vi "HighLvCtrl_Loop_Squat.vi"(8 "error in (no error)":errorcluster, 11 "HighLvClasses":T4={"CAlexVersion"=enum."Mobile", "CAlex2 out"=refnum, "ForceField"=refnum}) -> (0 "error out":errorcluster)   [LabVIEW 2016]
uses:
  <vilib>/Platform/TimedLoop/XDataNode/wakeup.ctl
  <vilib>/Platform/TimedLoop/XDataNode/XDNodeRunTimeDep.lvlib
  <vilib>/Platform/TimedLoop/XDataNode/nitl_modes.ctl
  <vilib>/Platform/TimedLoop/XDataNode/timing_clust.ctl
  <vilib>/Platform/TimedLoop/XDataNode/XDataNode.xnode
  Classes/SerialChain/SerialChain.lvclass
  Classes/SerialChain-Cable/SerialChain-Cable.lvclass
  Classes/ForceField/ForceField.lvclass
  <vilib>/Analysis/NI_AALBase.lvlib
  <vilib>/Analysis/Matrix/Datatypes/RealMatrix.ctl
  <vilib>/Analysis/Matrix/NI_Matrix.lvlib
  <vilib>/AuZn/auzn custom VIs/AuZnCustomVI.lvlib
  Classes/CAlex2/CAlex2.lvclass
  TypeDef/IMU_operation.ctl
  <vilib>/Analysis/baseanly.llb/A x Vector.vi
  C:/Users/randh/Desktop/BILATERAL/CAlex2-controller/Classes/SerialChain-Cable/SerialChain-Cable.lvclass
  C:/Users/randh/Desktop/BILATERAL/CAlex2-controller/Classes/SerialChain/SerialChain.lvclass
  Classes/ForceField/TypeDef/FF_Gains.ctl
  Classes/CAlex2/TypeDef/LowerBodyDim.ctl
  Classes/MotorControl/TypeDef/ControllerMode.ctl
  TypeDef/HighLvControl Cluster.ctl
  Classes/CAlex2/TypeDef/CAlexVersion.ctl
panel:
  in  "Use Vicon2JointAngle2 ?":bool=TRUE
  in  "Use IMU2JointAngle2 ?":bool=TRUE
  in  "history length (50)":i32=50
  in  "LP":bool=TRUE
  out "QPSolved":bool
  out "Torque Error":dbl[](array[numeric]) format="%#.4f"
  out "Torque":T1(graph)
  out "Joint Angles (deg)":T2(graph)
  out "Desired Torque":dbl[](array[numeric]) format="%#.4f"
  out "Actual Torque":dbl[](array[numeric]) format="%#.4f"
  in  "LockedJoints":i32[](array[numeric])=[2, 1]
  out "Jacobian for Cables":T3 format="%#.3f"
  in  "TargetF(N)":dbl=10.0 format="%#_13g"
  in  "LP fc":dbl=4.0 format="%0.3f"
  in  "QPmode":enum16{"tight", "loose", "adv"}(ring)=enum."adv"
  in  "F range":cluster{"Fmin":dbl, "Fmax":dbl}[](array[cluster])=[{"Fmin"=10.0, "Fmax"=80.0}, {"Fmin"=10.0, "Fmax"=80.0}, {"Fmin"=11.0, "Fmax"=80.0}, {"Fmin"=11.0, "Fmax"=80.0}]
  # "In Cable Order, Not Motor Order"
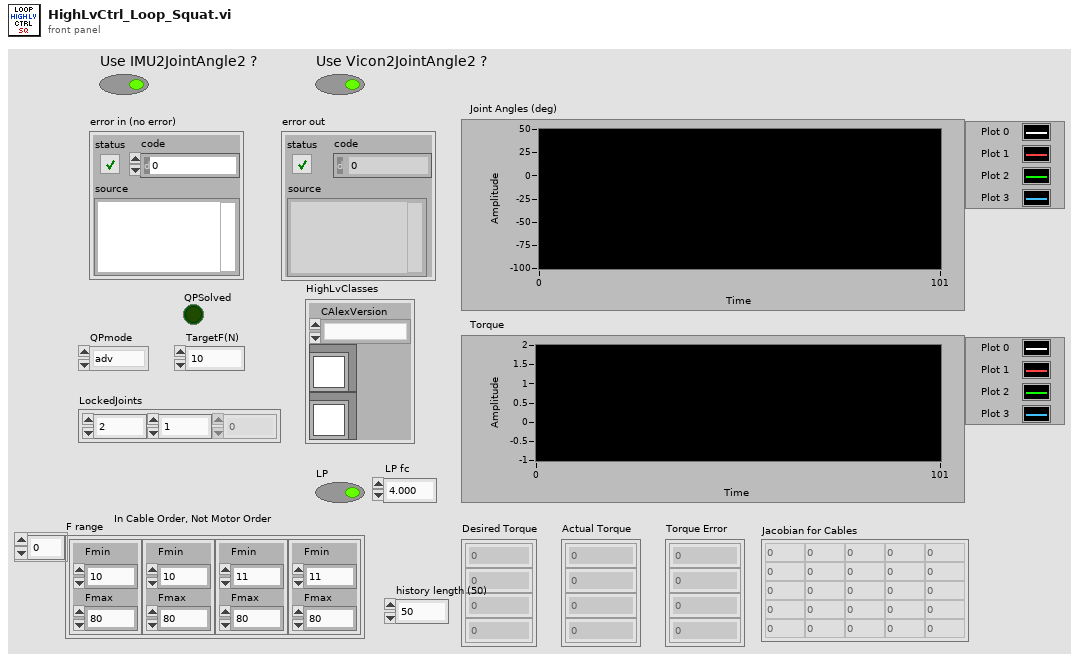
[diagram p1: front panel]
types:
  T1 = cluster{"[0]":dbl, "[1]":dbl, "[2]":dbl, "[3]":dbl, "[4]":dbl, "[5]":dbl, "[6]":dbl, "[7]":dbl, "[8]":dbl}
  T2 = cluster{"Joint Angles (rad)[0]":dbl, "Joint Angles (rad)[1]":dbl, "Joint Angles (rad)[2]":dbl, "Joint Angles (rad)[3]":dbl}
  T3 = typedef "NI_Matrix.lvlib/RealMatrix.ctl" = dbl[][]
  T4 = typedef "HighLvControl Cluster.ctl" = cluster{"CAlexVersion":T5, "CAlex2 out":refnum<class "CAlex2.lvclass">, "ForceField":refnum<class "ForceField.lvclass">}
  T5 = typedef "CAlex2.lvclass/CAlexVersion.ctl" = enum16{"Bilateral", "Squat", "Bilateral_Squat", "Treadmill", "Mobile"}
  T6 = typedef "XDNodeRunTimeDep.lvlib/timing_clust.ctl" = cluster{"Expected End [f-1]":u64, "Actual End [f-1]":u64, "Finished Late? [f-1]":bool, "Expected End [i-1]":u64, "Actual End [i-1]":u64, "Finished Late? [i-1]":bool, "Expected Start [i]":u64, "Actual Start [i]":u64, "Expected Start [f]":u64, "Actual Start [f]":u64, "Source Name":string, "Structure Name":string, "Period":i64, "Deadline":i64, "Offset":i64, "Start":i64, "Priority":i32, "Timeout":i32, "Mode":T7, "Wakeup Reason":T8, "Error":errorcluster, "Source Type":string, "Secondary Source Type":string, "Global End Time":u64, "Global Start Time":u64, "Frame Duration":u64, "Iteration Duration":u64, "Assigned CPU":i32, "I/O Scan Engine Mode":u32}
  T7 = typedef "XDNodeRunTimeDep.lvlib/nitl_modes.ctl" = enum32{"No Change", "Process missed periods, maintain original phase", "Discard missed periods, maintain original phase", "Process missed periods, ignore original phase", "Discard missed periods, ignore original phase"}
  T8 = typedef "XDNodeRunTimeDep.lvlib/wakeup.ctl" = enum32{"Normal", "Aborted", "Asynchronous wakeup", "Timing source error", "Timed loop error", "Timeout"}
  T9 = typedef "IMU_operation.ctl" = enum16{"GetData", "ClearStandPos", "SetStandPos"}
  T10 = typedef "ForceField.lvclass/FF_Gains.ctl" = cluster{"Kn":dbl, "Dn":dbl, "Kt":dbl, "Dt":dbl, "Kd":dbl, "Ns":dbl}
  T11 = typedef "CAlex2.lvclass/LowerBodyDim.ctl" = cluster{"BodyDim":cluster{"ThighLt (m)":dbl, "ShankLt (m)":dbl, "HipWd (m)":dbl}, "BodyWt":cluster{"Thigh (kg)":dbl, "Shank (kg)":dbl}, "Cuff Loc":cluster{"HipCuffWd (m)":dbl, "HipCuffHt (m)":dbl, "HipFwdShift (m)":dbl, "ThighToKnee (m)":dbl, "ThighCuffDist (m)":dbl, "ShankToKnee (m)":dbl}}
  T12 = typedef "SerialChain.lvclass/PointOnBody.ctl" = cluster{"Coord4":dbl[], "ID":i32}
  T13 = typedef "MotorControl.lvclass/ControllerMode.ctl" = enum16{"Idle", "FF", "PID"}
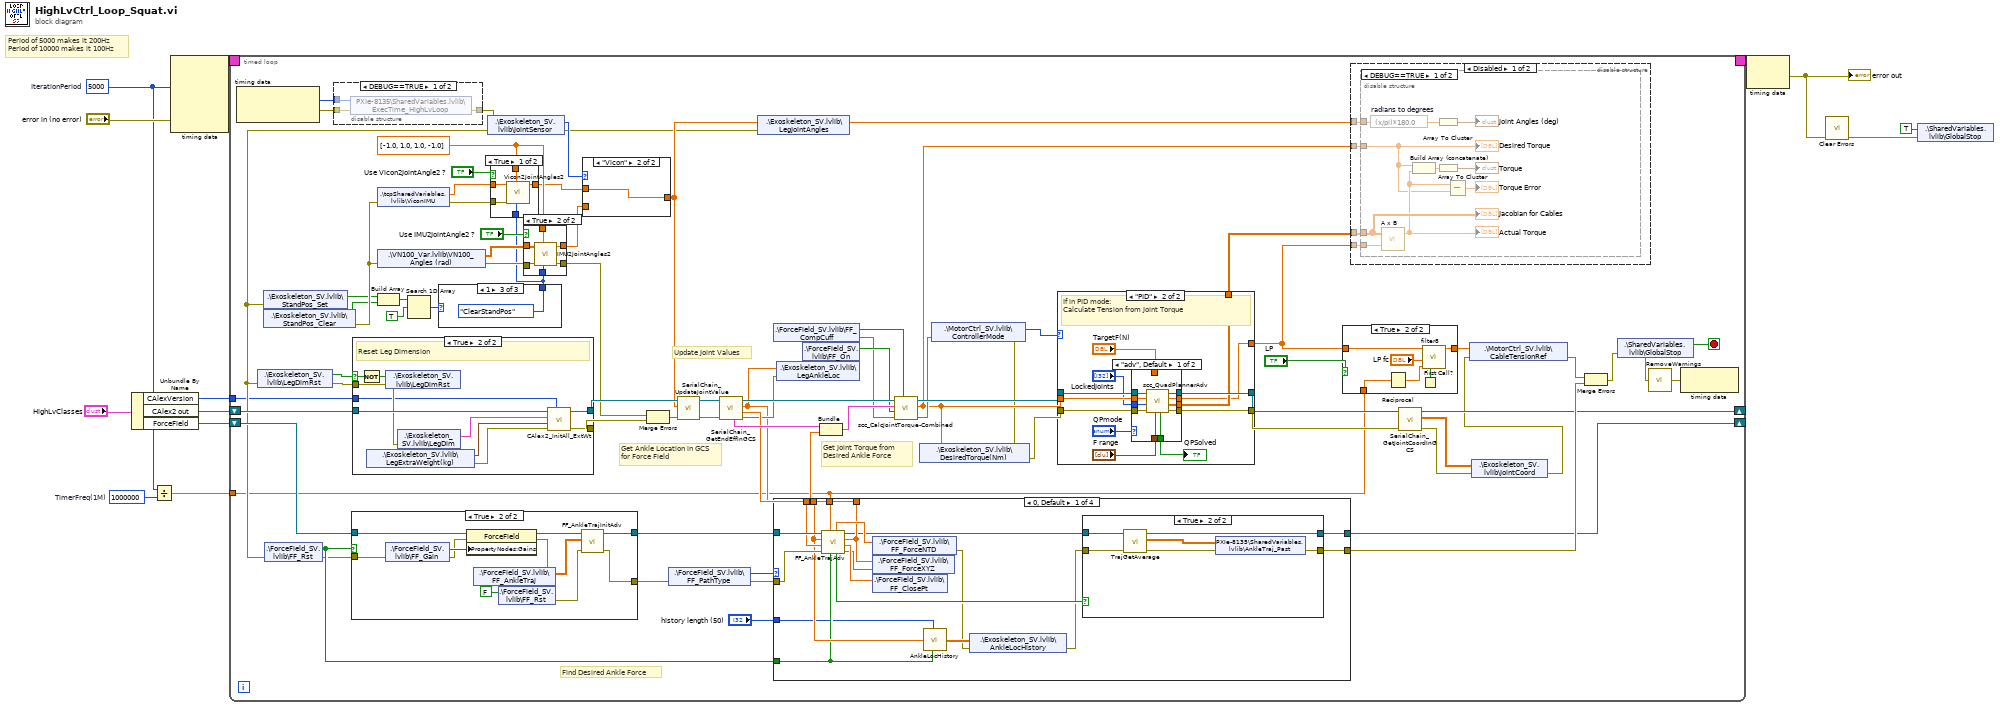
[diagram p0: block diagram]
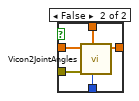
[diagram p5: hidden frame]
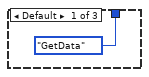
[diagram p6: hidden frame]
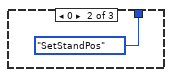
[diagram p7: hidden frame]
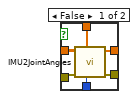
[diagram p8: hidden frame]
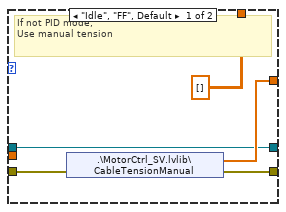
[diagram p11: hidden frame]
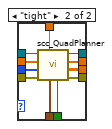
[diagram p12: hidden frame]
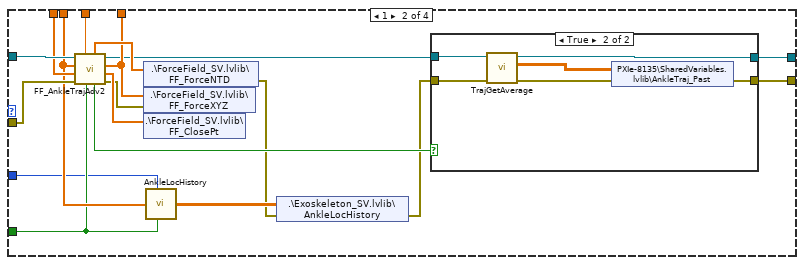
[diagram p16: hidden frame]
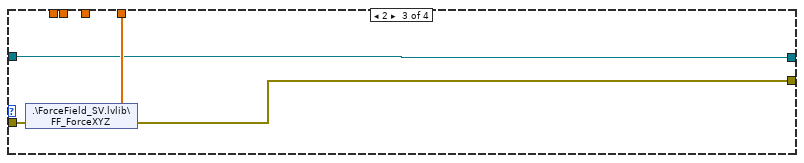
[diagram p18: hidden frame]
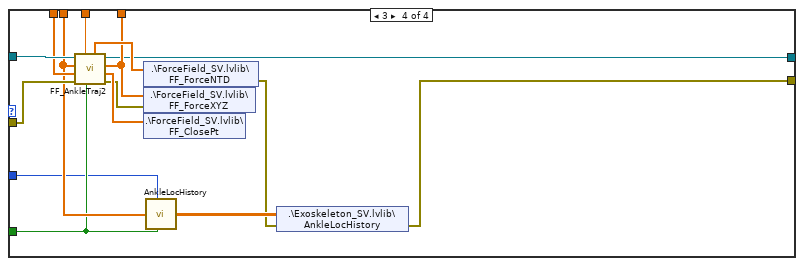
[diagram p19: hidden frame]
diagram:
  w3 = i64 1000000  # TimerFreq(1M)
  w4 = i64 5000  # IterationPeriod
  # "Period of 5000 makes it 200Hz\nPeriod of 10000 makes it 100Hz"
  n1 = Unbundle By Name("HighLvClasses") -> ("CAlexVersion"=w1:T5, "CAlex2 out"=w9:refnum<class "CAlex2.lvclass">, "ForceField"=w8:refnum<class "ForceField.lvclass">)
  n2 = Divide(x=w4, y=w3) -> (x/y=w2:dbl)
  n3 = node-c288(w4, "error in (no error)") -> (w13:T6)  [unwired: 3 in]
  n4 = timed-loop {
    timing: w13 -> [_]
    timing-out: [_] -> w12
    shift-right: [w47] -> _
    shift-left: w9 -> [w90]
    shift-right: [w60] -> _
    shift-left: w8 -> [w87]
    tunnel: w2 -> [w15]
    tunnel: w1 -> [w14]
    stop <- w62 stop-if-true
    w33 = dbl[] [-1.0, 1.0, 1.0, -1.0]
    # "Get Joint Torque from Desired Ankle Force"
    # "Find Desired Ankle Force"
    # "Get Ankle Location in GCS for Force Field"
    # "Update Joint Values"
    n5 = node-c288() -> (w89:i64, w88:errorcluster)  [unwired: 1 in]
    n6 = disable-structure shown="DEBUG==TRUE" {
      disable-tunnel: w89 -> [w141 _]
      disable-tunnel: w88 -> [w140 w142]
      disable-tunnel: [w139 w142] -> w17
      frame condition #0 {
        n7 = shared-variable "PXIe-8135\\SharedVariables.lvlib\\ExecTime_HighLvLoop"(w141, error in=w140) -> (error out=w139:errorcluster)
      }
      frame condition #1 (active) {
      }
    }
    n8 = shared-variable ".\\Exoskeleton_SV.lvlib\\LegDimRst"(error in=w17) -> (w71:bool, error out=w82:errorcluster)
    n9 = shared-variable ".\\Exoskeleton_SV.lvlib\\StandPos_Set"(error in=w17) -> (w25:bool, error out=w64:errorcluster)
    n10 = shared-variable ".\\Exoskeleton_SV.lvlib\\StandPos_Clear"(error in=w64) -> (w24:bool, error out=w32:errorcluster)
    n11 = shared-variable ".\\ForceField_SV.lvlib\\FF_Rst"(error in=w17) -> (w68:bool, error out=w67:errorcluster)
    n12 = case shown="True" w68 {
      tunnel: w87 -> [w182 w194]
      tunnel: [w182 w193] -> w81
      tunnel: w67 -> [w181 w189]
      tunnel: [w181 w183] -> w70
      frame False {
      }
      frame True {
        n13 = shared-variable ".\\ForceField_SV.lvlib\\FF_Gain"(error in=w189) -> (w192:T10, error out=w187:errorcluster)
        n14 = property class="ForceField"(reference=w194, error in=w187, "PropertyNodes:Gains"=w192) -> (reference out=w191:refnum<class "ForceField.lvclass">, error out=w186:errorcluster)
        n15 = shared-variable ".\\ForceField_SV.lvlib\\FF_AnkleTraj"(error in=w186) -> (w190:dbl[][], error out=w185:errorcluster)
        n16 = shared-variable ".\\ForceField_SV.lvlib\\FF_Rst"(FALSE ("FFRst"), error in=w185) -> (error out=w184:errorcluster)
        n17 = call "FF_AnkleTrajInitAdv.vi"("error in (no error)"=w184, "AnkleTraj"=w190, "Force Field Controller in"=w191) -> ("error out"=w183:errorcluster, "Force Field Controller out"=w193:refnum<class "ForceField.lvclass">)  [unwired: 6 in, 1 out]
      }
    }
    n18 = case shown="True" w71 {
      selector: w71 -> [_ w203]
      tunnel: w90 -> [w196 w208]
      tunnel: [w196 w207] -> w83
      tunnel: w82 -> [w195 w206]
      tunnel: [w195 w201] -> w39
      tunnel: w14 -> [_ w197]
      frame False {
      }
      frame True {
        # "Reset Leg Dimension"
        n19 = Not(x=w203) -> (.not. x?=w204:bool)
        n20 = shared-variable ".\\Exoskeleton_SV.lvlib\\LegDimRst"(w204, error in=w206) -> (error out=w200:errorcluster)
        n21 = shared-variable ".\\Exoskeleton_SV.lvlib\\LegDim"(error in=w200) -> (w205:T11, error out=w199:errorcluster)
        n22 = shared-variable ".\\Exoskeleton_SV.lvlib\\LegExtraWeight(kg)"(error in=w199) -> (w202:cluster{"Thigh":dbl, "Shank":dbl}, error out=w198:errorcluster)
        n23 = call "CAlex2_InitAll_ExtWt.vi"("CAlexVersion"=w197, "error in (no error)"=w198, "ExtraWeight(kg)"=w202, "LegProperties"=w205, "CAlex2 in"=w208) -> ("error out"=w201:errorcluster, "CAlex2 out"=w207:refnum<class "CAlex2.lvclass">)  [unwired: 5 in]
      }
    }
    n24 = shared-variable ".\\VN100_Var.lvlib\\VN100_Angles (rad)"(error in=w32) -> (w36:dbl[][], error out=w37:errorcluster)
    n25 = Build Array(w25, w24) -> (w23:bool[])
    n26 = shared-variable ".\\tcpSharedVariables.lvlib\\ViconIMU"(error in=w32) -> (w35:dbl[], error out=w34:errorcluster)
    n27 = Search 1D Array(1D array=w23, element=TRUE) -> (index of element=w22:i32)  [unwired: 1 in]
    n28 = case shown="1" w22 {
      tunnel: [IMU_operation."GetData" ("Operation(GetData)") IMU_operation."SetStandPos" ("Operation(GetData)") IMU_operation."ClearStandPos" ("Operation(GetData)")] -> w20
      frame Default {
      }
      frame 0 {
      }
      frame 1 {
      }
    }
    n29 = shared-variable ".\\Exoskeleton_SV.lvlib\\JointSensor"(error in=w17) -> (w31:enum16{"IMU", "Vicon"}, error out=w27:errorcluster)
    n30 = case shown="True" "Use Vicon2JointAngle2 ?" {
      tunnel: w35 -> [w116 w121]
      tunnel: w34 -> [w115 w120]
      tunnel: w33 -> [w114 w119]
      tunnel: [w113 w118] -> w30
      tunnel: w20 -> [w112 w117]
      frame True {
        n31 = call "Vicon2JointAngles2.vi"("Operation(GetData)"=w112, "JointAngleDir([-1,1,1,-1])"=w114, "error in (no error)"=w115, "ViconIMU in (rad)"=w116) -> ("Joint Angles (rad)"=w113:dbl[])  [unwired: 6 in, 1 out]
      }
      frame False {
        n32 = call "Vicon2JointAngles.vi"("Operation(GetData)"=w117, "JointAngleDir([-1,1,1,-1])"=w119, "error in (no error)"=w120, "ViconIMU in (rad)"=w121) -> ("Joint Angles (rad)"=w118:dbl[])  [unwired: 6 in, 1 out]
      }
    }
    n33 = case shown="True" "Use IMU2JointAngle2 ?" {
      tunnel: w37 -> [w130 w136]
      tunnel: w36 -> [w129 w135]
      tunnel: w33 -> [w128 w134]
      tunnel: [w127 w133] -> w29
      tunnel: w20 -> [w126 w132]
      tunnel: [w125 w131] -> w19
      frame False {
        n34 = call "IMU2JointAngles.vi"("Operation(GetData)"=w126, "JointAngleDir (-1, 1, 1,-1)"=w128, "error in (no error)"=w130, "IMU in (rad)"=w129) -> ("error out"=w125:errorcluster, "Joint Angles (rad)"=w127:dbl[])  [unwired: 6 in]
      }
      frame True {
        n35 = call "IMU2JointAngles2.vi"("Operation(GetData)"=w132, "JointAngleDir (-1, 1, 1,-1)"=w134, "error in (no error)"=w136, "IMU in (rad)"=w135) -> ("error out"=w131:errorcluster, "Joint Angles (rad)"=w133:dbl[])  [unwired: 6 in]
      }
    }
    n36 = case shown="\"Vicon\"" w31 {
      tunnel: w30 -> [_ w138]
      tunnel: [w137 w138] -> w28
      tunnel: w29 -> [w137 _]
      frame "IMU", Default {
      }
      frame "Vicon" {
      }
    }
    n37 = Merge Errors(w19, w39) -> (w38:errorcluster)
    n38 = shared-variable ".\\ForceField_SV.lvlib\\FF_PathType"(error in=w70) -> (w77:i8, error out=w76:errorcluster)
    n39 = call "SerialChain_UpdateJointValue.vi"("error in (no error)"=w38, "JointAngle (rad | m)"=w28, "SerialChain in"=w83) -> ("error out"=w50:errorcluster, "SerialChain out"=w51:refnum<class "CAlex2.lvclass">)  [unwired: 7 in]
    n40 = call "SerialChain_GetEndEffInGCS.vi"("error in (no error)"=w50, "SerialChain in"=w51) -> ("error out"=w69:errorcluster, "Vendeff(GCS)"=w78:dbl[], "Pendeff(GCS)"=w43:dbl[], "SerialChain out"=w85:refnum<class "CAlex2.lvclass">, "EndEffPos"=w86:T12)  [unwired: 5 in]
    n41 = shared-variable ".\\Exoskeleton_SV.lvlib\\LegJointAngles"(w28, error in=w27) -> ()  [unwired: 1 out]
    n42 = case shown="0, Default" w77 {
      tunnel: w81 -> [w228 w256 w267 w285]
      tunnel: w76 -> [w224 w252 w266 w281]
      tunnel: [w217 w245 w267 w271] -> w60
      tunnel: [w223 w251 w268 w280] -> w79
      tunnel: w43 -> [w213 w241 _ w274]
      tunnel: w78 -> [w220 w248 _ w277]
      tunnel: w15 -> [w219 w247 _ w276]
      tunnel: w68 -> [w212 w240 _ w273]
      tunnel: [w216 w244 w265 w270] -> w61
      tunnel: "history length (50)" -> [w209 w237 _ w269]
      frame 0, Default {
        n43 = call "FF_AnkleTrajAdv.vi"("Init"=w212, "dt"=w219, "error in (no error)"=w224, "AnkleVelocity"=w220, "AnkleInGCS"=w213, "Force Field Controller in"=w228) -> ("error out"=w222:errorcluster, "ClosestPoint"=w226:dbl[], "ForceXYZ"=w223:dbl[], "Force Field Controller out"=w218:refnum<class "ForceField.lvclass">, "UpdateTrajPrev"=w215:bool, "ForceNTD"=w227:dbl[])
        n44 = shared-variable ".\\ForceField_SV.lvlib\\FF_ForceXYZ"(w223, error in=w222) -> (error out=w221:errorcluster)
        n45 = shared-variable ".\\ForceField_SV.lvlib\\FF_ClosePt"(w226, error in=w221) -> (error out=w225:errorcluster)
        n46 = shared-variable ".\\ForceField_SV.lvlib\\FF_ForceNTD"(w227, error in=w225) -> (error out=w211:errorcluster)
        n47 = call "AnkleLocHistory.vi"("history length (100)"=w209, "AnkleLoc"=w213, "initialize"=w212) -> ("AnkleLoc"=w214:dbl[][])  [unwired: 2 in]
        n48 = shared-variable ".\\Exoskeleton_SV.lvlib\\AnkleLocHistory"(w214, error in=w211) -> (error out=w210:errorcluster)
        n49 = case shown="True" w215 {
          tunnel: w218 -> [w230 w235]
          tunnel: [w230 w236] -> w217
          tunnel: w210 -> [w229 w233]
          tunnel: [w229 w231] -> w216
          frame False {
          }
          frame True {
            n50 = call-dynamic "TrajGetAverage.vi"("error in (no error)"=w233, "ForceField in"=w235) -> ("error out"=w232:errorcluster, "Ankle Traj Ave"=w234:dbl[][], "ForceField out"=w236:refnum<class "ForceField.lvclass">)  [unwired: 7 in]
            n51 = shared-variable "PXIe-8135\\SharedVariables.lvlib\\AnkleTraj_Past"(w234, error in=w232) -> (error out=w231:errorcluster)
          }
        }
      }
      frame 1 {
        n52 = call "FF_AnkleTrajAdv2.vi"("Init"=w240, "dt"=w247, "error in (no error)"=w252, "AnkleVelocity"=w248, "AnkleInGCS"=w241, "Force Field Controller in"=w256) -> ("error out"=w250:errorcluster, "ClosestPoint"=w254:dbl[], "Assistive Force in GCS"=w251:dbl[], "Force Field Controller out"=w246:refnum<class "ForceField.lvclass">, "UpdateTrajAve"=w243:bool, "Assistive Force FnFtFd"=w255:dbl[])
        n53 = shared-variable ".\\ForceField_SV.lvlib\\FF_ForceXYZ"(w251, error in=w250) -> (error out=w249:errorcluster)
        n54 = shared-variable ".\\ForceField_SV.lvlib\\FF_ClosePt"(w254, error in=w249) -> (error out=w253:errorcluster)
        n55 = shared-variable ".\\ForceField_SV.lvlib\\FF_ForceNTD"(w255, error in=w253) -> (error out=w239:errorcluster)
        n56 = call "AnkleLocHistory.vi"("history length (100)"=w237, "AnkleLoc"=w241, "initialize"=w240) -> ("AnkleLoc"=w242:dbl[][])  [unwired: 2 in]
        n57 = shared-variable ".\\Exoskeleton_SV.lvlib\\AnkleLocHistory"(w242, error in=w239) -> (error out=w238:errorcluster)
        n58 = case shown="True" w243 {
          tunnel: w246 -> [w258 w263]
          tunnel: [w258 w264] -> w245
          tunnel: w238 -> [w257 w261]
          tunnel: [w257 w259] -> w244
          frame False {
          }
          frame True {
            n59 = call-dynamic "TrajGetAverage.vi"("error in (no error)"=w261, "ForceField in"=w263) -> ("error out"=w260:errorcluster, "Ankle Traj Ave"=w262:dbl[][], "ForceField out"=w264:refnum<class "ForceField.lvclass">)  [unwired: 7 in]
            n60 = shared-variable "PXIe-8135\\SharedVariables.lvlib\\AnkleTraj_Past"(w262, error in=w260) -> (error out=w259:errorcluster)
          }
        }
      }
      frame 2 {
        n61 = shared-variable ".\\ForceField_SV.lvlib\\FF_ForceXYZ"(error in=w266) -> (w268:dbl[], error out=w265:errorcluster)
      }
      frame 3 {
        n62 = call "FF_AnkleTraj2.vi"("Init"=w273, "dt"=w276, "error in (no error)"=w281, "AnkleVelocity"=w277, "AnkleInGCS"=w274, "Force Field Controller in"=w285) -> ("error out"=w279:errorcluster, "ClosePt"=w283:dbl[], "Force"=w280:dbl[], "Force Field Controller out"=w271:refnum<class "ForceField.lvclass">, "ForceComp"=w284:dbl[])  [unwired: 1 in]
        n63 = shared-variable ".\\ForceField_SV.lvlib\\FF_ForceXYZ"(w280, error in=w279) -> (error out=w278:errorcluster)
        n64 = shared-variable ".\\ForceField_SV.lvlib\\FF_ClosePt"(w283, error in=w278) -> (error out=w282:errorcluster)
        n65 = shared-variable ".\\ForceField_SV.lvlib\\FF_ForceNTD"(w284, error in=w282) -> (error out=w272:errorcluster)
        n66 = call "AnkleLocHistory.vi"("history length (100)"=w269, "AnkleLoc"=w274, "initialize"=w273) -> ("AnkleLoc"=w275:dbl[][])  [unwired: 2 in]
        n67 = shared-variable ".\\Exoskeleton_SV.lvlib\\AnkleLocHistory"(w275, error in=w272) -> (error out=w270:errorcluster)
      }
    }
    n68 = shared-variable ".\\Exoskeleton_SV.lvlib\\LegAnkleLoc"(w43, error in=w69) -> (error out=w74:errorcluster)
    n69 = shared-variable ".\\ForceField_SV.lvlib\\FF_On"(error in=w74) -> (w73:bool, error out=w75:errorcluster)
    n70 = shared-variable ".\\ForceField_SV.lvlib\\FF_CompCuff"(error in=w75) -> (w59:bool, error out=w72:errorcluster)
    n71 = Bundle("EndEffPos"=w86, "Force"=w79) -> (w80:cluster{"EndEffPos":T12, "Force":dbl[]})  [unwired: 1 in]
    n72 = call "scc_CalcJointTorque-Combined.vi"("CuffWtComp?(T)"=w59, "error in (no error)"=w72, "ExternalForce(T)"=w73, "External Force (In GCS)"=w80, "SerialChain_Cable in"=w85) -> ("error out"=w56:errorcluster, "DesiredTorque(Nm)"=w42:dbl[], "SerialChain_Cable out"=w84:refnum<class "CAlex2.lvclass">)  [unwired: 4 in]
    n73 = shared-variable ".\\MotorCtrl_SV.lvlib\\ControllerMode"(error in=w56) -> (w57:T13, error out=w41:errorcluster)
    n74 = shared-variable ".\\Exoskeleton_SV.lvlib\\DesiredTorque(Nm)"(w42, error in=w41) -> (error out=w40:errorcluster)
    n75 = case shown="\"PID\"" w57 {
      tunnel: [w146 w159] -> w49
      tunnel: w40 -> [w145 w158]
      tunnel: w84 -> [w146 w157]
      tunnel: [T3 [] ("Jacobian for Cables") w153] -> w66
      tunnel: w42 -> [_ w152]
      tunnel: [w147 w151] -> w58
      tunnel: [w144 w150] -> w48
      frame "Idle", "FF", Default {
        # "If not PID mode,\nUse manual tension"
        n76 = shared-variable ".\\MotorCtrl_SV.lvlib\\CableTensionManual"(error in=w145) -> (w147:dbl[], error out=w144:errorcluster)
      }
      frame "PID" {
        # "If in PID mode:\nCalculate Tension from Joint Torque"
        n77 = case shown="\"adv\", Default" "QPmode" {
          tunnel: w158 -> [w162 w180]
          tunnel: w157 -> [w168 w179]
          tunnel: w152 -> [w167 w172]
          tunnel: [w169 w178] -> w159
          tunnel: "F range" -> [w164 w177]
          tunnel: [w163 w176] -> w156
          tunnel: [w166 w175] -> w151
          tunnel: [w165 w174] -> w150
          tunnel: "TargetF(N)" -> [_ w173]
          tunnel: "LockedJoints" -> [w161 w171]
          tunnel: [w160 w170] -> w153
          frame "adv", Default {
            n78 = call "scc_QuadPlannerAdv.vi"("F range (of each cable)"=w164, "error in (no error)"=w162, "LockedJoint(StartFrom0)"=w161, "DesireTorque(Nm)"=w167, "SerialChain_Cable in"=w168) -> ("error out"=w165:errorcluster, "Jacobian for Cables"=w160:T3, "Planned Tension"=w166:dbl[], "SerialChain_Cable out"=w169:refnum<class "CAlex2.lvclass">, "Solved"=w163:bool)  [unwired: 2 in]
          }
          frame "tight" {
            n79 = call "scc_QuadPlanner.vi"("F range"=w177, "TargetF(N)"=w173, "error in (no error)"=w180, "LockedJoint(StartFrom0)"=w171, "DesireTorque(Nm)"=w172, "SerialChain_Cable in"=w179) -> ("error out"=w174:errorcluster, "Jacobian for Cables"=w170:T3, "Planned Tension"=w175:dbl[], "SerialChain_Cable out"=w178:refnum<class "CAlex2.lvclass">, "Solved"=w176:bool)  [unwired: 1 in]
          }
        }
        "QPSolved" <- w156
      }
    }
    n80 = case shown="True" "LP" {
      tunnel: w58 -> [w91 w95]
      tunnel: [w91 w94] -> w55
      tunnel: w15 -> [_ w92]
      frame False {
      }
      frame True {
        n81 = Reciprocal(x=w92) -> (1/x=w96:dbl)
        n82 = First Call?() -> (First Call?: T/F=w93:bool)
        n83 = call "filter8.vi"("initialize"=w93, "sampling freq: fs"=w96, "low cutoff freq: fl"="LP fc", "X"=w95) -> ("Filtered X"=w94:dbl[])  [unwired: 7 in]
      }
    }
    n84 = disable-structure shown="Disabled" {
      disable-tunnel: w66 -> [w101 _]
      disable-tunnel: w58 -> [w100 _]
      disable-tunnel: w42 -> [w99 _]
      disable-tunnel: w28 -> [w98 _]
      frame Disabled {
        n85 = disable-structure shown="DEBUG==TRUE" {
          disable-tunnel: w101 -> [w111 _]
          disable-tunnel: w100 -> [w110 _]
          disable-tunnel: w98 -> [w109 _]
          disable-tunnel: w99 -> [w103 _]
          frame condition #0 {
            n86 = expression code="(x/pi)*180.0" "radians to degrees"(w109) -> (w106:dbl[])
            n87 = call-poly <vilib>:"A x B.vi"("Vector"=w110, "A"=w111) -> ("A x Vector"=w104:dbl[])  [unwired: 1 out]
            "Actual Torque" <- w104
            n88 = Build Array (concatenate)(w103, w104) -> (w107:dbl[])
            n89 = Array To Cluster(array=w106) -> (cluster=→"Joint Angles (deg)":T2)
            n90 = Array To Cluster(array=w107) -> (cluster=→"Torque":T1)
            n91 = Subtract(x=w104, y=w103) -> (x-y=→"Torque Error":dbl[])
            "Jacobian for Cables" <- w111
            "Desired Torque" <- w103
          }
          frame condition #1 (active) {
          }
        }
      }
      frame Enabled {
      }
    }
    n92 = call "SerialChain_GetJointCoordInGCS.vi"("error in (no error)"=w48, "SerialChain in"=w49) -> ("error out"=w45:errorcluster, "Joint Coord in GCS"=w46:dbl[][], "SerialChain out"=w47:refnum<class "CAlex2.lvclass">)  [unwired: 5 in, 2 out]
    n93 = shared-variable ".\\Exoskeleton_SV.lvlib\\JointCoord"(w46, error in=w45) -> (error out=w44:errorcluster)
    n94 = shared-variable ".\\MotorCtrl_SV.lvlib\\CableTensionRef"(w55, error in=w44) -> (error out=w65:errorcluster)
    n95 = Merge Errors(w65, w61) -> (w63:errorcluster)
    n96 = shared-variable ".\\SharedVariables.lvlib\\GlobalStop"(error in=w63) -> (w62:bool, error out=w54:errorcluster)
    n97 = call <vilib>:"RemoveWarnings.vi"("error in (no error)"=w54) -> ("error out"=w53:errorcluster)
    n98 = node-c288(w53) -> ()  [unwired: 1 out]
  }
  n99 = node-c288(w12) -> (w6:errorcluster)
  "error out" <- w6
  n100 = call <vilib>:"Clear Errors.vi"("error in (no error)"=w6) -> ("error out"=w5:errorcluster)  [unwired: 5 in, 1 out]
  n101 = shared-variable ".\\SharedVariables.lvlib\\GlobalStop"(TRUE ("GlobalStop"), error in=w5) -> ()  [unwired: 1 out]
